vi "Step5.vi"() -> ()   [LabVIEW 2025]
uses:
  <vilib>/Analysis/5stat.llb/RMS (DBL).vi
  <vilib>/Utility/file.llb/Read Delimited Spreadsheet (DBL).vi
  <vilib>/express/express analysis/Spectral/Block/exnSpectralBlock spectral measurements peak poly.vi
  <vilib>/express/express analysis/Spectral/Block/exnSpectralBlock spectral measurements peak DDT.vi
  <vilib>/express/express analysis/Spectral/XNode/ExpressSpectralMeasurementsBlockNode.xnode
  <vilib>/Analysis/NI_AALBase.lvlib
  <vilib>/Analysis/NI_AAL_SigProc.lvlib
  <vilib>/Analysis/NI_AALPro.lvlib
panel:
  out "rms value":dbl format="%0.2f"
  out "Signal Representation":dbl[](graph)
  out "Amplitudes":dbl[](array[numeric])
  out "Frequency":dbl[](array[numeric])
  out "Fourier Analysis":dynamicdata(graph)
  out "Filtered Signal":dynamicdata(graph)
  out "After Outlier Removal":waveform(dbl)(graph)
  in  "Z Threshold":dbl
  in  "Data File Path":path
  out "Time vs Signal":waveform(dbl)(graph)
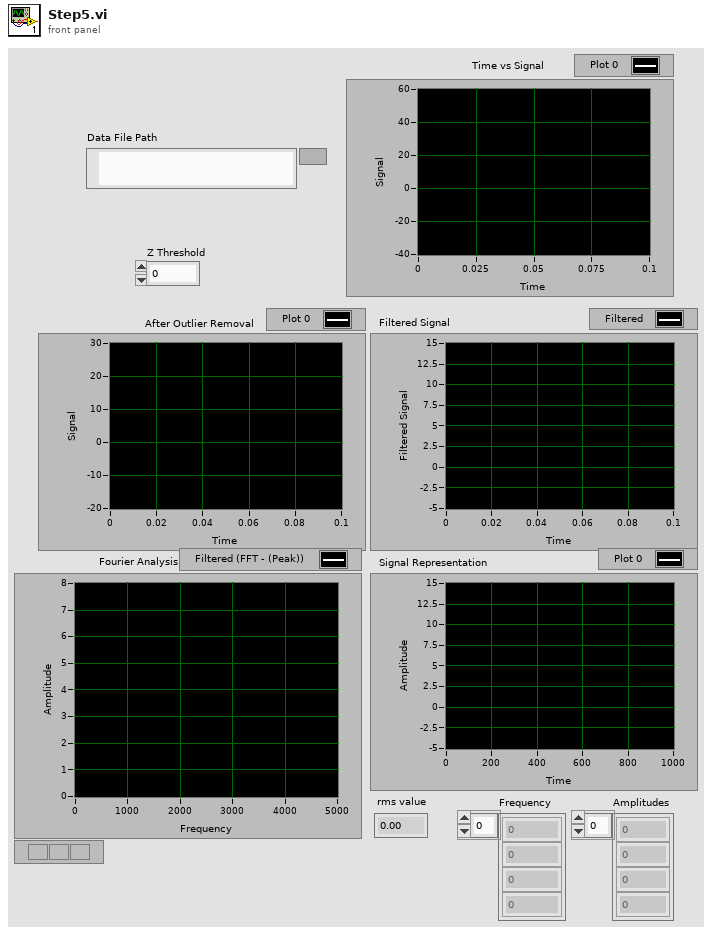
[diagram p1: front panel]
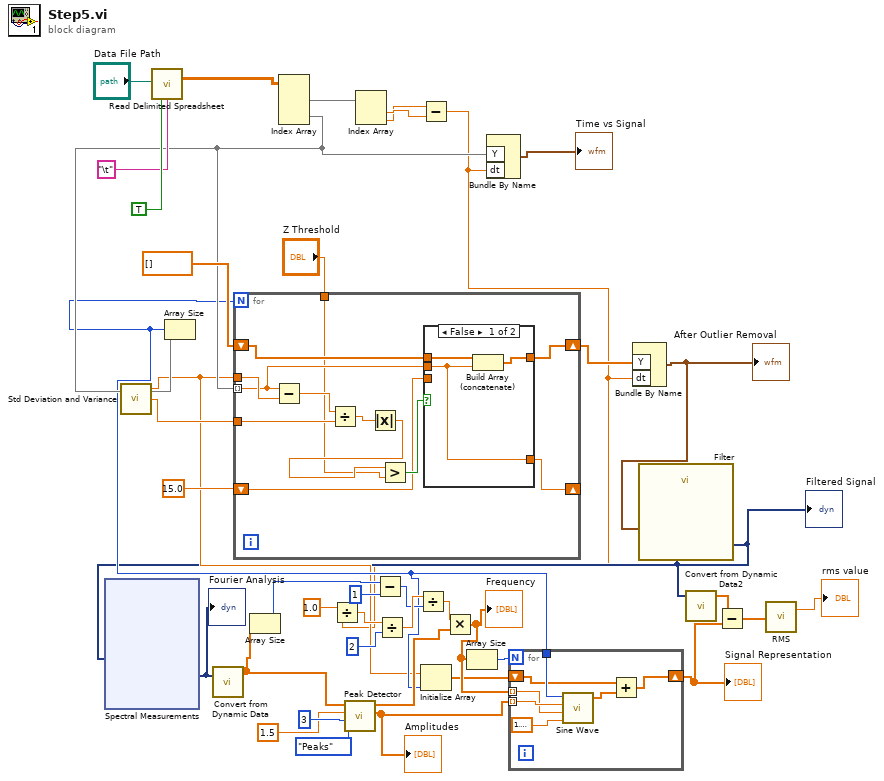
[diagram p0: block diagram]
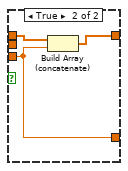
[diagram p2: hidden frame]
diagram:
  n1 = call-poly <vilib>:"Read Delimited Spreadsheet.vi"("file path (dialog if empty)"="Data File Path", "transpose? (F)"=TRUE, "delimiter (\\t)"="\t" ("delimiter (\\t)")) -> ("all rows"=w39:dbl[][])  [unwired: 7 in, 5 out]
  n2 = Index Array(array=w39) -> (element #1=w38:dbl[], element #2=w28:dbl[])  [unwired: 4 in]
  n3 = call <vilib>:"Std Deviation and Variance.vi"("X"=w28) -> ("mean"=w7:dbl, "standard deviation"=w33:dbl)  [unwired: 1 in, 1 out]
  n4 = Array Size(array=w28) -> (size(s)=w9:i32)
  n5 = for {
    N: w9 -> [_]
    shift-right: [w48] -> w30
    tunnel: w33 -> [w52]
    tunnel: w28 -> [w46] mode=indexing
    tunnel: w7 -> [w50]
    tunnel: "Z Threshold" -> [w42]
    shift-left: dbl[] [] -> [w47]
    shift-right: [w44] -> _
    shift-left: 15.0 -> [w45]
    n6 = Subtract(x=w46, y=w50) -> (x-y=w53:dbl)
    n7 = Divide(x=w53, y=w52) -> (x/y=w51:dbl)
    n8 = Absolute Value(x=w51) -> (abs(x)=w43:dbl)
    n9 = Greater?(x=w43, y=w42) -> (0:w49:bool)
    n10 = case shown="False" w49 {
      tunnel: w46 -> [w54 _]
      tunnel: w47 -> [w55 w59]
      tunnel: [w56 w58] -> w48
      tunnel: w45 -> [_ w57]
      tunnel: [w54 w57] -> w44
      frame False {
        n11 = Build Array (concatenate)(w55, w54) -> (w56:dbl[])
      }
      frame True {
        n12 = Build Array (concatenate)(w59, w57) -> (w58:dbl[])
      }
    }
  }
  n13 = Index Array(array=w38) -> (element #1=w37:dbl, element #2=w29:dbl)  [unwired: 2 in]
  n14 = Subtract(x=w29, y=w37) -> (x-y=w1:dbl)
  n15 = Divide(x=1.0, y=w1) -> (x/y=w19:dbl)
  n16 = Divide(x=w19, y=2) -> (x/y=w17:dbl)
  n17 = Initialize Array(w7, w9) -> (w8:dbl[])
  n18 = Bundle By Name("Y"=w28, "dt"=w1) -> (→"Time vs Signal":waveform(dbl))  [unwired: 1 in]
  n19 = Bundle By Name("Y"=w30, "dt"=w1) -> (w27:waveform(dbl))  [unwired: 1 in]
  "After Outlier Removal" <- w27
  n20 = call "Filter"("Signal"=w27) -> ("Filtered Signal"=w6:dynamicdata)  [unwired: 9 in, 1 out]
  "Filtered Signal" <- w6
  n21 = xnode "Spectral Measurements"("Signals"=w6) -> ("FFT - (Peak)"=w23:dynamicdata)  [unwired: 1 in, 2 out]
  "Fourier Analysis" <- w23
  n22 = call "Convert from Dynamic Data"("Dynamic Data Type"=w23) -> ("Array"=w22:dbl[])  [unwired: 3 in]
  n23 = Array Size(array=w22) -> (size(s)=w15:i32)
  n24 = call <vilib>:"Peak Detector.vi"("peaks/valleys"=enum32{"Peaks", "Valleys"}."Peaks", "width"=3, "threshold"=1.5, "X"=w22) -> ("Amplitudes"=w11:dbl[], "Locations"=w14:dbl[])  [unwired: 3 in, 3 out]
  "Amplitudes" <- w11
  n25 = Subtract(x=w15, y=1) -> (x-y=w16:i32)
  n26 = Divide(x=w17, y=w16) -> (x/y=w13:dbl)
  n27 = Multiply(x=w13, y=w14) -> (x*y=w10:dbl[])
  "Frequency" <- w10
  n28 = Array Size(array=w10) -> (size(s)=w12:i32)
  n29 = for {
    N: w12 -> [_]
    tunnel: w11 -> [w65] mode=indexing
    tunnel: w10 -> [w64] mode=indexing
    tunnel: w9 -> [w63]
    shift-right: [w60] -> w4
    shift-left: w8 -> [w61]
    n30 = call <vilib>:"Sine Wave.vi"("samples"=w63, "amplitude"=w65, "frequency"=w64, "phase in"=1.5707963267948966) -> ("sine wave"=w62:dbl[])  [unwired: 1 in, 2 out]
    n31 = Add(x=w61, y=w62) -> (x+y=w60:dbl[])
  }
  "Signal Representation" <- w4
  n32 = call "Convert from Dynamic Data2"("Dynamic Data Type"=w6) -> ("Array"=w5:dbl[])  [unwired: 3 in]
  n33 = Subtract(x=w5, y=w4) -> (x-y=w3:dbl[])
  n34 = call-poly <vilib>:"RMS.vi"("X"=w3) -> ("rms value"=→"rms value":dbl)  [unwired: 1 out]
